vi "Get Value (JSON).vi"(8 "error in (no error)":errorcluster, 10 "key":string, 11 "JSON Value in":refnum<class "JSON Value.lvclass">) -> (0 "error out":errorcluster, 2 "JSON Value out":refnum<class "JSON Value.lvclass">)   [LabVIEW 2016, in "JSON Value.lvclass"]
uses:
  JSON Value.lvclass
  JSON Value.lvclass/JSON Value.ctl
  subVIs/Errors.ctl
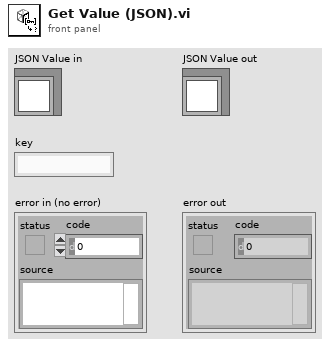
[diagram p1: front panel]
types:
  T1 = typedef "JSON Value.lvclass/Errors.ctl" = enum16{"No key", "Key path type", "Array OOB", "Type Mismatch", "Invalid Token"}
  T2 = typedef "JSON Value.lvclass/JSON Types.ctl" = enum16{"String", "Numeric", "Boolean", "NULL", "Object", "Array"}
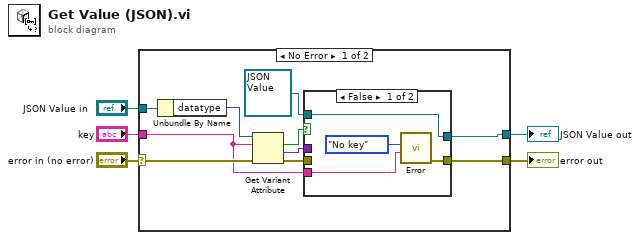
[diagram p0: block diagram]
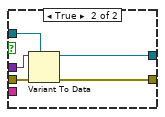
[diagram p2: hidden frame]
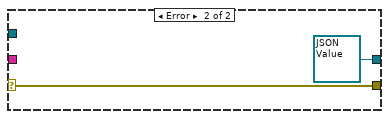
[diagram p3: hidden frame]
diagram:
  n1 = case shown="No Error" "error in (no error)" {
    selector: "error in (no error)" -> [w13 w26]
    tunnel: [w11 w26] -> w4
    tunnel: "JSON Value in" -> [w15 _]
    tunnel: "key" -> [w7 _]
    tunnel: [w10 refnum<class "JSON Value.lvclass"> refnum ("JSON Helper.lvclass")] -> w1
    frame No Error {
      n2 = Unbundle By Name(w15) -> ("datatype"=w9:T2)
      n3 = Get Variant Attribute(Variant=w9, name=w7, error in=w13) -> (found=w8:bool, value=w14:variant, error out=w12:errorcluster)  [unwired: 1 in, 1 out]
      n4 = case shown="False" w8 {
        tunnel: w14 -> [_ w24]
        tunnel: w12 -> [_ w23]
        tunnel: [w18 w22] -> w11
        tunnel: refnum<class "JSON Value.lvclass"> refnum ("JSON Helper.lvclass") -> [w19 w21]
        tunnel: [w19 w20] -> w10
        tunnel: w7 -> [w16 _]
        frame False {
          n5 = call "Error.vi"("Data"=w16, 9:Errors."No key") -> ("error out"=w18:errorcluster)  [unwired: 8 in]
        }
        frame True {
          n6 = Variant To Data(error in=w23, type=w21, Variant=w24) -> (data=w20:refnum<class "JSON Value.lvclass">, error out=w22:errorcluster)
        }
      }
    }
    frame Error {
    }
  }
  "error out" <- w4
  "JSON Value out" <- w1
